vi "System judgment voltage.vi"(7 "Voltage":dbl, 11 "Temperature":dbl) -> (2 "Voltage 2":dbl, 3 "Voltage 1":dbl)   [LabVIEW 2019, in "nematic.lvlib" / "Copy of StrainCell.lvlib"]
uses:
  Copy of StrainCell.lvlib
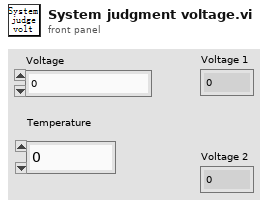
[diagram p1: front panel]
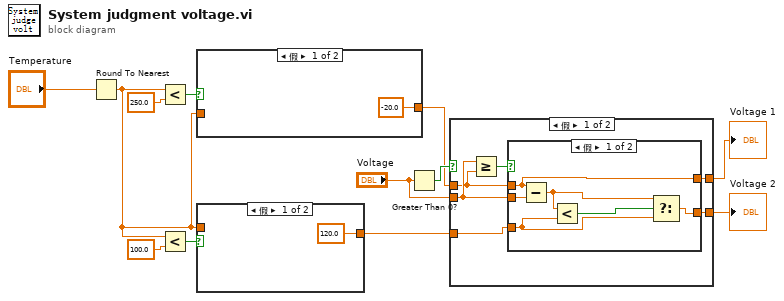
[diagram p0: block diagram]
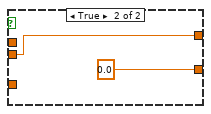
[diagram p2: hidden frame]
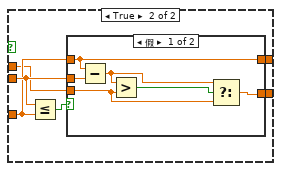
[diagram p3: hidden frame]
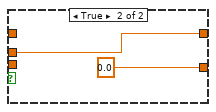
[diagram p4: hidden frame]
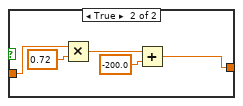
[diagram p5: hidden frame]
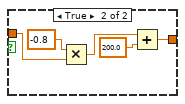
[diagram p6: hidden frame]
diagram:
  n1 = Round To Nearest(number="Temperature") -> (nearest integer value=w7:dbl)
  n2 = Less?(x=w7, y=250.0) -> (x < y?=w8:bool)
  n3 = Less?(x=w7, y=100.0) -> (x < y?=w10:bool)
  n4 = case shown="假" w8 {
    tunnel: w7 -> [_ w18]
    tunnel: [-20.0 w14] -> w1
    frame False {
    }
    frame True {
      n5 = Multiply(x=w18, y=0.72) -> (x*y=w16:dbl)
      n6 = Add(x=w16, y=-200.0) -> (x+y=w14:dbl)
    }
  }
  n7 = case shown="假" w10 {
    tunnel: w7 -> [_ w21]
    tunnel: [120.0 w20] -> w6
    frame False {
    }
    frame True {
      n8 = Multiply(x=-0.8, y=w21) -> (x*y=w23:dbl)
      n9 = Add(x=w23, y=200.0) -> (x+y=w20:dbl)
    }
  }
  n10 = Greater Than 0?(x="Voltage") -> (x > 0?=w5:bool)
  n11 = case shown="假" w5 {
    tunnel: w6 -> [w25 w42]
    tunnel: "Voltage" -> [w29 w43]
    tunnel: w1 -> [w26 w39]
    tunnel: [w27 w41] -> w3
    tunnel: [w28 w40] -> w2
    frame False {
      n12 = Greater Or Equal?(x=w29, y=w26) -> (x >= y?=w30:bool)
      n13 = case shown="假" w30 {
        tunnel: w29 -> [w35 w38]
        tunnel: [w36 w38] -> w28
        tunnel: [w32 0.0 ("Voltage 2")] -> w27
        tunnel: w26 -> [w36 _]
        tunnel: w25 -> [w33 _]
        frame False {
          n14 = Subtract(x=w36, y=w35) -> (x-y=w34:dbl)
          n15 = Less?(x=w34, y=w33) -> (x < y?=w31:bool)
          n16 = Select(t=w34, s=w31, f=w33) -> (s? t:f=w32:dbl)
        }
        frame True {
        }
      }
    }
    frame True {
      n17 = Less Or Equal?(x=w43, y=w42) -> (x <= y?=w44:bool)
      n18 = case shown="假" w44 {
        tunnel: w43 -> [w49 w52]
        tunnel: [w50 w52] -> w40
        tunnel: [w46 0.0 ("Voltage 2")] -> w41
        tunnel: w42 -> [w50 _]
        tunnel: w39 -> [w47 _]
        frame False {
          n19 = Subtract(x=w50, y=w49) -> (x-y=w48:dbl)
          n20 = Greater?(x=w48, y=w47) -> (0:w45:bool)
          n21 = Select(t=w48, s=w45, f=w47) -> (s? t:f=w46:dbl)
        }
        frame True {
        }
      }
    }
  }
  "Voltage 1" <- w2
  "Voltage 2" <- w3
